vi "Create Sequence.vi"(8 "error in (no error)":errorcluster, 11 "QPA Measurement in":refnum<class "QPA Measurement.lvclass">) -> (0 "error out":errorcluster, 3 "QPA Measurement out":refnum<class "QPA Measurement.lvclass">)   [LabVIEW 2016, in "QPA Measurement.lvlib" / "QPA Measurement.lvclass"]
uses:
  QPA Measurement.lvclass
  C:/Projects/STS/Common/Sequence Automation/Plugins/Measurement Interface.lvlibp/Measurement Interface.lvclass
  QPA Measurement.lvclass/QPA Measurement.ctl
  Protected Methods/Read Measurement Name.vi
  Plugins/Measurement Interface.lvlibp/Private Methods/Engine Reference/Read Engine Reference.vi
  Plugins/Measurement Interface.lvlibp/Private Methods/Active Sequence File/Read Active Sequence File.vi
  Plugins/TestStand API Tools (TSAT).lvlibp/Sequence Actions/TSAT Sequence Actions.lvlib
  Plugins/TestStand API Tools (TSAT).lvlibp/Sequence File Actions/TSAT Sequence File Actions.lvlib
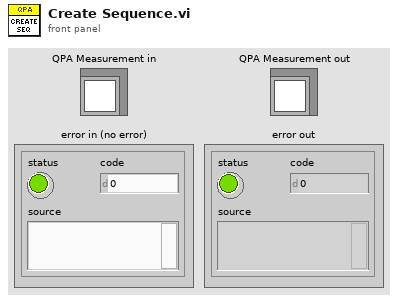
[diagram p1: front panel]
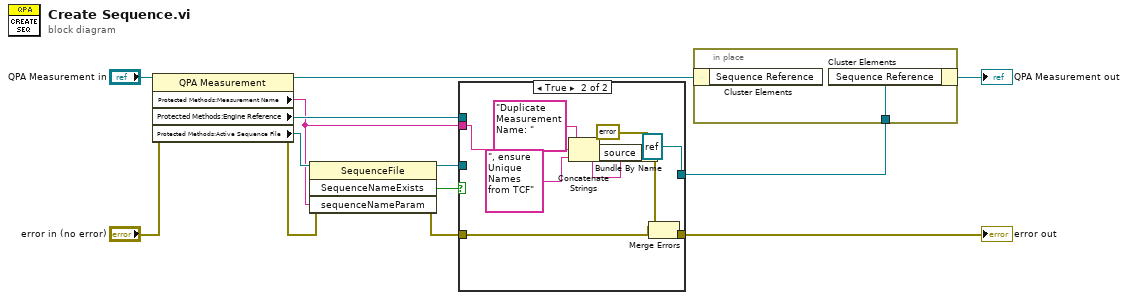
[diagram p0: block diagram]
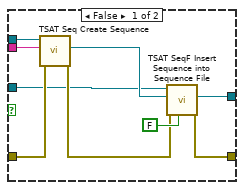
[diagram p2: hidden frame]
diagram:
  n1 = property class="QPA Measurement"(reference="QPA Measurement in", error in="error in (no error)") -> (reference out=w11:refnum<class "QPA Measurement.lvclass">, error out=w6:errorcluster, "Protected Methods:Measurement Name"=w2:string, "Protected Methods:Engine Reference"=w10:refnum<k7>, "Protected Methods:Active Sequence File"=w4:refnum<k7>)
  n2 = invoke class="SequenceFile" method="SequenceNameExists"(reference=w4, error in=w6, "sequenceNameParam"=w2) -> (reference out=w3:refnum<k7>, error out=w5:errorcluster, "SequenceNameExists"=w1:bool)  [unwired: 1 in, 1 out]
  n3 = case shown="True" w1 {
    tunnel: [w22 refnum<k7> refnum ("Sequence Reference Out")] -> w12
    tunnel: w10 -> [w20 _]
    tunnel: [w19 w24] -> w9
    tunnel: w5 -> [w16 w23]
    tunnel: w3 -> [w15 _]
    tunnel: w2 -> [w14 w27]
    frame False {
      n4 = call "TSAT Seq Create Sequence.vi"("Error in"=w16, "Sequence Name"=w14, "Engine In"=w20) -> ("Error out"=w18:errorcluster, "Sequence Reference Out"=w17:refnum<k7>)  [unwired: 6 in, 1 out]
      n5 = call "TSAT SeqF Insert Sequence into Sequence File.vi"("Close Sequence Reference?(T)"=FALSE, "Error in"=w18, "Sequence to Insert"=w17, "Sequence File"=w15) -> ("Error Out"=w19:errorcluster, "Sequence Reference Out"=w22:refnum<k7>)  [unwired: 5 in, 1 out]
    }
    frame True {
      n6 = Concatenate Strings("Duplicate Measurement Name: ", w27, ", ensure Unique Names from TCF" ("string")) -> (w29:string)
      n7 = Bundle By Name(cluster=errorcluster {"status"=TRUE, "code"=8354, "source"=""} ("error constant"), "source"=w29) -> (w30:errorcluster)
      n8 = Merge Errors(w23, w30) -> (w24:errorcluster)
    }
  }
  "error out" <- w9
  n9 = in-place {
    in-place-border: w12 -> [w32]
    n10 = in-place-cluster #1(w11) -> ()  [unwired: 1 out]
    n11 = in-place-cluster #1("Sequence Reference"=w32) -> (→"QPA Measurement out":refnum<class "QPA Measurement.lvclass">)
  }
